vi "insert_example.vi"   [LabVIEW 2020, in "Data.PG.lvclass"]
uses:
  Data.PG.lvclass
types:
  T1 = cluster{"host":string, "port":string, "dbname":string, "user":string, "password":string}
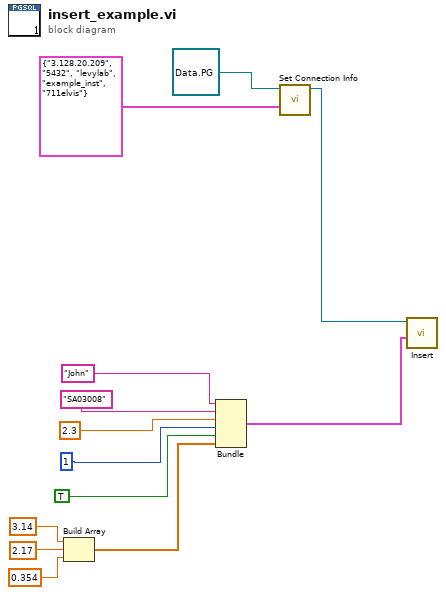
[diagram p0: block diagram]
diagram:
  n1 = Build Array(3.14, 2.17, 0.354) -> (w9:dbl[])
  n2 = Bundle("John", "SA03008", 2.3, 1, TRUE, w9) -> (w2:cluster{string, string, dbl, i32, bool, dbl[]})  [unwired: 1 in]
  n3 = call "Set Connection Info.vi"("connection info"=T1 {"host"="3.128.20.209", "port"="5432", "dbname"="levylab", "user"="example_inst", "password"="711elvis"}, "Data.PG in"=refnum<class "Data.PG.lvclass"> refnum) -> ("Data.PG out"=w6:refnum<class "Data.PG.lvclass">)  [unwired: 8 in, 1 out]
  n4 = call "Insert.vi"("Data"=w2, "Data.PG in"=w6) -> ()  [unwired: 8 in, 2 out]
